vi "Helicopter - Config Dialog.vi"(8 "error in (no error)":errorcluster, 10 "In":T1, 11 "NIVS.System Definition Root":refnum<k24>) -> (0 "error out":errorcluster, 2 "Out":T1)   [LabVIEW 2014]
uses:
  Data.ctl
  NationalInstruments.VeriStand.SystemStorageUI
  NationalInstruments.VeriStand.SystemStorage
  <vilib>/NI Veristand/UI Controls/Single Node Browser/NI_VS UI Single Node Browser.lvlib
panel:
  in  "Travel":refnum<k24>(container)
  in  "Pitch":refnum<k24>(container)
  in  "Elevation":refnum<k24>(container)
  in  "Cancel":bool
  in  "Ok":bool
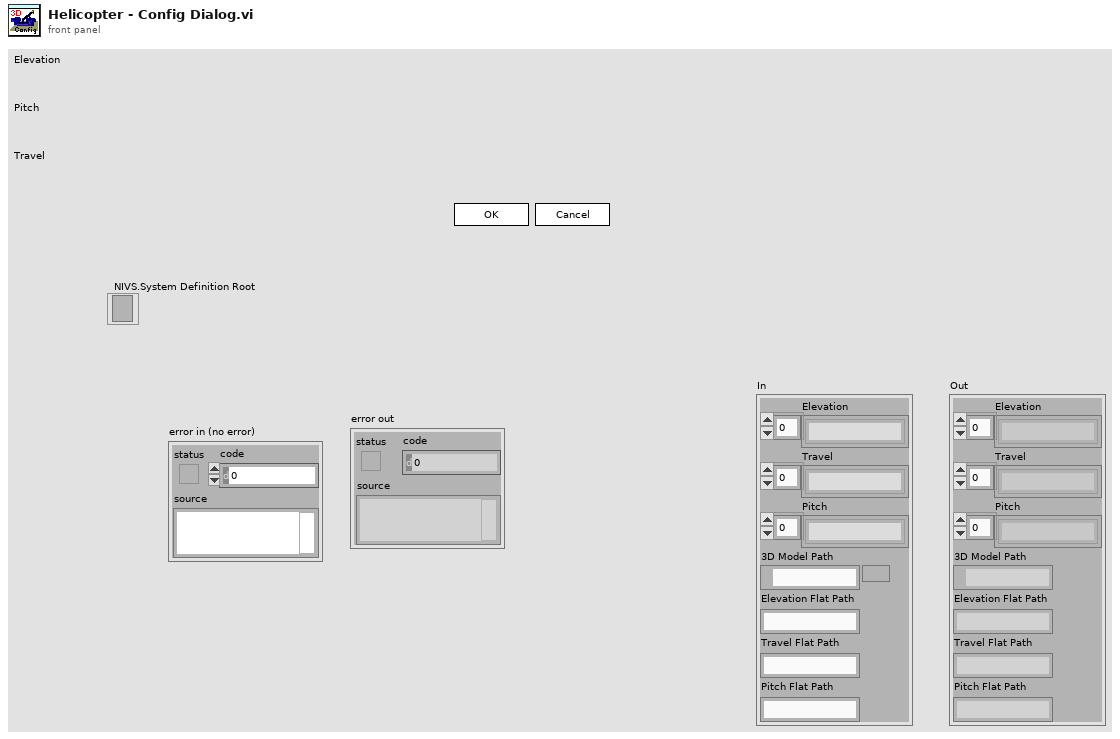
[diagram p1: front panel]
types:
  T1 = typedef "Data.ctl" = cluster{"Elevation":string[], "Travel":string[], "Pitch":string[], "3D Model Path":path, "Elevation Flat Path":string, "Travel Flat Path":string, "Pitch Flat Path":string}
  T2 = typedef "NI_VS UI Single Node Browser.lvlib/Callback Type.ctl" = cluster{"Net Callbacks":refnum<k27>[], "Event":refnum<user-event>}
  T3 = typedef "NI_VS UI Single Node Browser.lvlib/Node Ref.ctl" = refnum<k24>
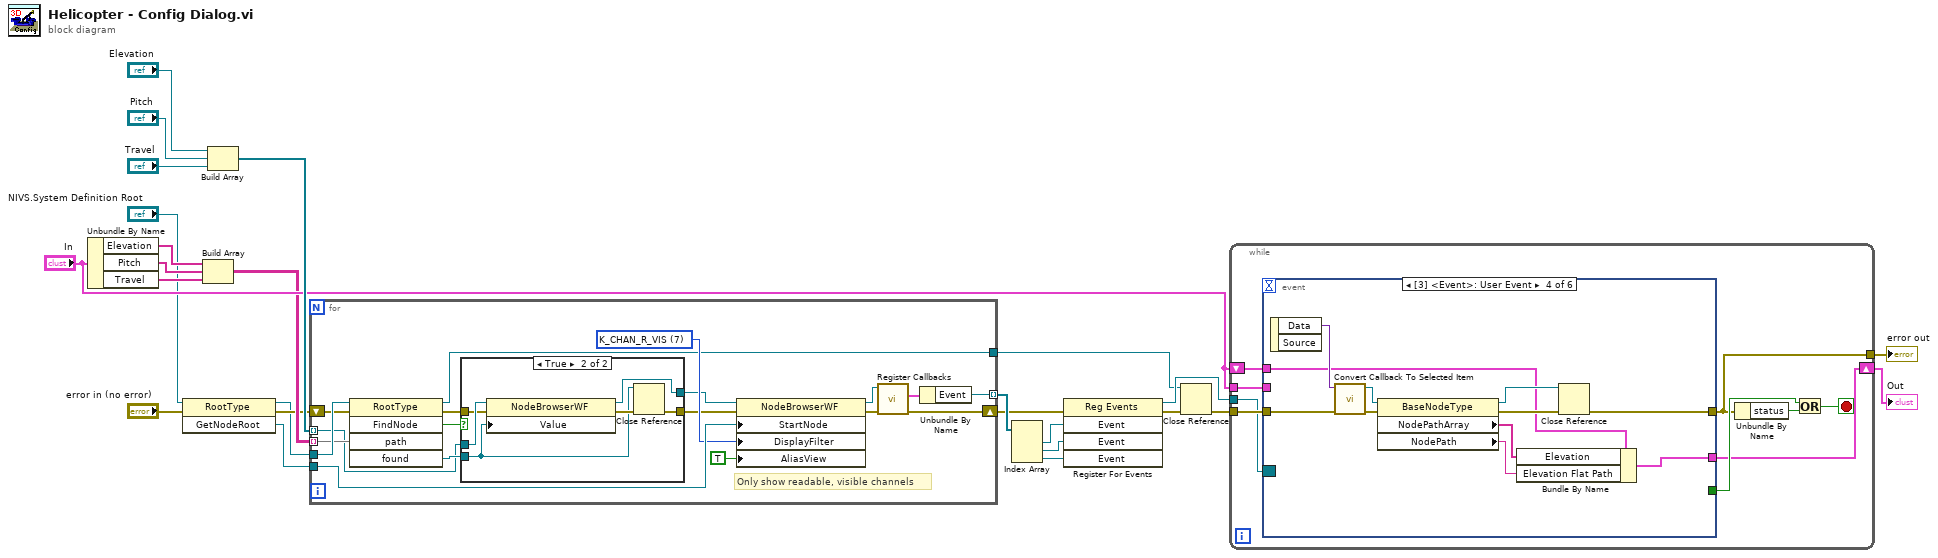
[diagram p0: block diagram]
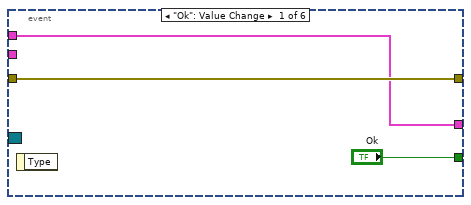
[diagram p3: hidden frame]
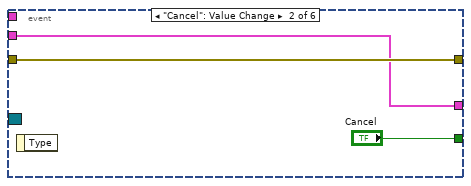
[diagram p4: hidden frame]
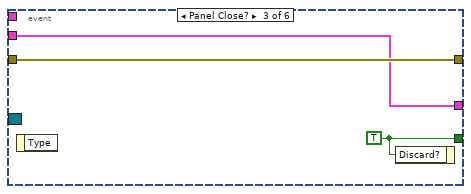
[diagram p5: hidden frame]
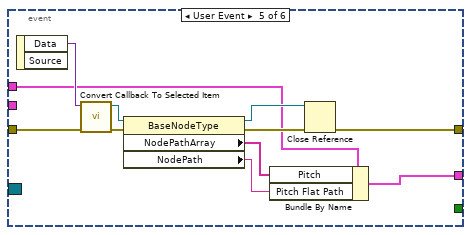
[diagram p6: hidden frame]
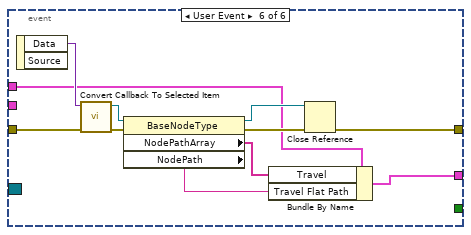
[diagram p7: hidden frame]
diagram:
  n1 = Unbundle By Name("In") -> ("Elevation"=w9:string[], "Pitch"=w10:string[], "Travel"=w11:string[])
  n2 = invoke class="RootType" method="GetNodeRoot"(reference="NIVS.System Definition Root", error in="error in (no error)") -> (reference out=w2:refnum<k24>, error out=w3:errorcluster, "GetNodeRoot"=w1:refnum<k24>)  [unwired: 1 in]
  n3 = Build Array(w9, w10, w11) -> (w8:string[][])
  n4 = Build Array("Elevation", "Pitch", "Travel") -> (w21:refnum<k24>[])
  n5 = for {
    tunnel: w21 -> [w28] mode=indexing
    tunnel: w1 -> [w41]
    shift-right: [w26] -> w16
    shift-left: w3 -> [w34]
    tunnel: [w37] -> w20 mode=indexing
    tunnel: w8 -> [w35] mode=indexing
    tunnel: w2 -> [w36]
    tunnel: [w30] -> w7
    w39 = u8 7 items=["K_CHAN_R", "K_CHAN_W", "K_CHAN_RW", "K_CHAN_VOLT", "K_CHAN_FAULT", "K_ALL", "K_CUSTOM", "K_CHAN_R_VIS", "K_CHAN_W_VIS", "K_CHAN_RW_VIS", "K_CHAN_VOLT_VIS", "K_CHAN_FAULT_VIS"] ("DisplayFilter")
    # "Only show readable, visible channels"
    n6 = invoke class="RootType" method="FindNode"(reference=w36, error in=w34, "path"=w35) -> (reference out=w30:refnum<k24>, error out=w32:errorcluster, "FindNode"=w29:bool, "found"=w33:refnum<k24>)  [unwired: 2 in, 1 out]
    n7 = case shown="True" w29 {
      tunnel: w33 -> [_ w46]
      tunnel: w32 -> [w45 w47]
      tunnel: [w45 w50] -> w31
      tunnel: w28 -> [w44 w49]
      tunnel: [w44 w48] -> w27
      frame False {
      }
      frame True {
        n8 = property class="NodeBrowserWF"(reference=w49, error in=w47, "Value"=w46) -> (reference out=w48:refnum<k24>, error out=w51:errorcluster)
        n9 = Close Reference(reference=w46, error in (no error)=w51) -> (error out=w50:errorcluster)
      }
    }
    n10 = property class="NodeBrowserWF"(reference=w27, error in=w31, "StartNode"=w41, "DisplayFilter"=w39, "AliasView"=TRUE) -> (reference out=w40:refnum<k24>, error out=w42:errorcluster)
    n11 = call <vilib>:"Register Callbacks.vi"("error in (no error)"=w42, "Single Node Browser"=w40) -> ("error out"=w26:errorcluster, "Callbacks"=w43:T2)  [unwired: 7 in, 1 out]
    n12 = Unbundle By Name(w43) -> ("Event"=w37:refnum<user-event>)
  }
  n13 = Index Array(array=w20) -> (element #1=w19:refnum<user-event>, element #2=w18:refnum<user-event>, element #3=w17:refnum<user-event>)  [unwired: 3 in]
  n14 = register-events(error in=w16, w19, w18, w17) -> (reference out=w14:refnum<event-registration>, error out=w15:errorcluster)  [unwired: 1 in]
  n15 = Close Reference(reference=w7, error in (no error)=w15) -> (error out=w4:errorcluster)
  n16 = while {
    tunnel: [w58] -> w25
    tunnel: w4 -> [w59]
    tunnel: w14 -> [w55]
    tunnel: "In" -> [w53]
    shift-right: [w54] -> w13
    shift-left: "In" -> [w52]
    stop <- w57 stop-if-true
    n17 = event shown="[3] <Event>: User Event" {
      selector: w55 -> [_ _ _ _ _ _]
      dyn-events: _ -> [_ _ _ _ _ _]
      timeout: _ -> [_ _ _ _ _ _]
      tunnel: ["Ok" "Cancel" w69 _ _ _] -> w60
      tunnel: [w63 w65 w68 w78 w89 w100] -> w58
      tunnel: w59 -> [w63 w65 w68 w79 w90 w101]
      tunnel: [w61 w64 w67 w71 w83 w94] -> w54
      tunnel: w53 -> [_ w64 w67 _ _ _]
      tunnel: w52 -> [w61 _ _ w73 w84 w95]
      event "Ok": Value Change {
        n18 = event-data() -> ()  [unwired: 1 in, 1 out]
      }
      event "Cancel": Value Change {
        n19 = event-data() -> ()  [unwired: 1 in, 1 out]
      }
      event Panel Close? {
        w69 = TRUE ("Cancel")
        n20 = event-data() -> ()  [unwired: 1 in, 1 out]
        n21 = event-data("Discard?"=w69) -> ()  [unwired: 1 in, 1 out]
      }
      event User Event {
        n22 = event-data() -> ("Data"=w80:variant)  [unwired: 1 in, 1 out]
        n23 = call <vilib>:"Convert Callback To Selected Item.vi"("error in"=w79, "Data"=w80) -> ("error out"=w74:errorcluster, "Selected Item"=w77:T3)  [unwired: 8 in]
        n24 = property class="BaseNodeType"(reference=w77, error in=w74) -> (reference out=w76:T3, error out=w75:errorcluster, "NodePathArray"=w72:string[], "NodePath"=w70:string)
        n25 = Bundle By Name(cluster=w73, "Elevation"=w72, "Elevation Flat Path"=w70) -> (w71:T1)
        n26 = Close Reference(reference=w76, error in (no error)=w75) -> (error out=w78:errorcluster)
      }
      event User Event {
        n27 = event-data() -> ("Data"=w91:variant)  [unwired: 1 in, 1 out]
        n28 = call <vilib>:"Convert Callback To Selected Item.vi"("error in"=w90, "Data"=w91) -> ("error out"=w85:errorcluster, "Selected Item"=w88:T3)  [unwired: 8 in]
        n29 = property class="BaseNodeType"(reference=w88, error in=w85) -> (reference out=w87:T3, error out=w86:errorcluster, "NodePathArray"=w82:string[], "NodePath"=w81:string)
        n30 = Bundle By Name(cluster=w84, "Pitch"=w82, "Pitch Flat Path"=w81) -> (w83:T1)
        n31 = Close Reference(reference=w87, error in (no error)=w86) -> (error out=w89:errorcluster)
      }
      event User Event {
        n32 = event-data() -> ("Data"=w102:variant)  [unwired: 1 in, 1 out]
        n33 = call <vilib>:"Convert Callback To Selected Item.vi"("error in"=w101, "Data"=w102) -> ("error out"=w96:errorcluster, "Selected Item"=w99:T3)  [unwired: 8 in]
        n34 = property class="BaseNodeType"(reference=w99, error in=w96) -> (reference out=w98:T3, error out=w97:errorcluster, "NodePathArray"=w93:string[], "NodePath"=w92:string)
        n35 = Bundle By Name(cluster=w95, "Travel"=w93, "Travel Flat Path"=w92) -> (w94:T1)
        n36 = Close Reference(reference=w98, error in (no error)=w97) -> (error out=w100:errorcluster)
      }
    }
    n37 = Unbundle By Name(w58) -> ("status"=w56:bool)
    n38 = Or(x=w60, y=w56) -> (x .or. y?=w57:bool)
  }
  "Out" <- w13
  "error out" <- w25
